vi "Read gRCP to Main.vi"(8 "error in (no error)":errorcluster, 11 "CIFTemplatePlugin in":refnum<class "TemplatePlugin.lvclass">) -> (0 "error out":errorcluster, 3 "CIFTemplatePlugin out":refnum<class "TemplatePlugin.lvclass">)   [LabVIEW 2021, in "TemplatePlugin.lvclass"]
uses:
  TemplatePlugin.lvclass
  TemplatePlugin.lvclass/TemplatePlugin.ctl
  CIF-LVCore/src/CIFUtilities/CIFOutOfBand/CIFOutOfBand.lvclass/CIFOutOfBand.ctl
  OOB/OOB_Rx/Private/Read Payload.vi
  CIF-LVCore/src/CIFUtilities/CIFOutOfBand/Read OOB DVR.vi
  OOB/OOB_Rx/Private/Command Settings.vi
  CIF-LVCore/src/CIFUtilities/CIFOutOfBand/Accessors/Read Local OOB Data.vi
  OOB/OOB_Rx/TemplateOOB_Rx.lvclass
  D:/dev/CIF-LVCore/src/CIFUtilities/CIFOutOfBand/CIFOutOfBand.lvclass
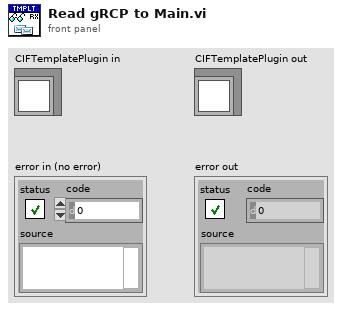
[diagram p1: front panel]
types:
  T1 = typedef "TemplateOOB_Rx.lvclass/OOB Commands.ctl" = enum8{"Command 1"}
  T2 = typedef "TemplateOOB_Rx.lvclass/gRPC to Main Command Data.ctl" = cluster{"Cmd 1 Data":i32}
  T3 = typedef "TemplatePlugin.lvclass/gRPC to Main Cyclic Data.ctl" = cluster{"Cyclic Data 1":i32}
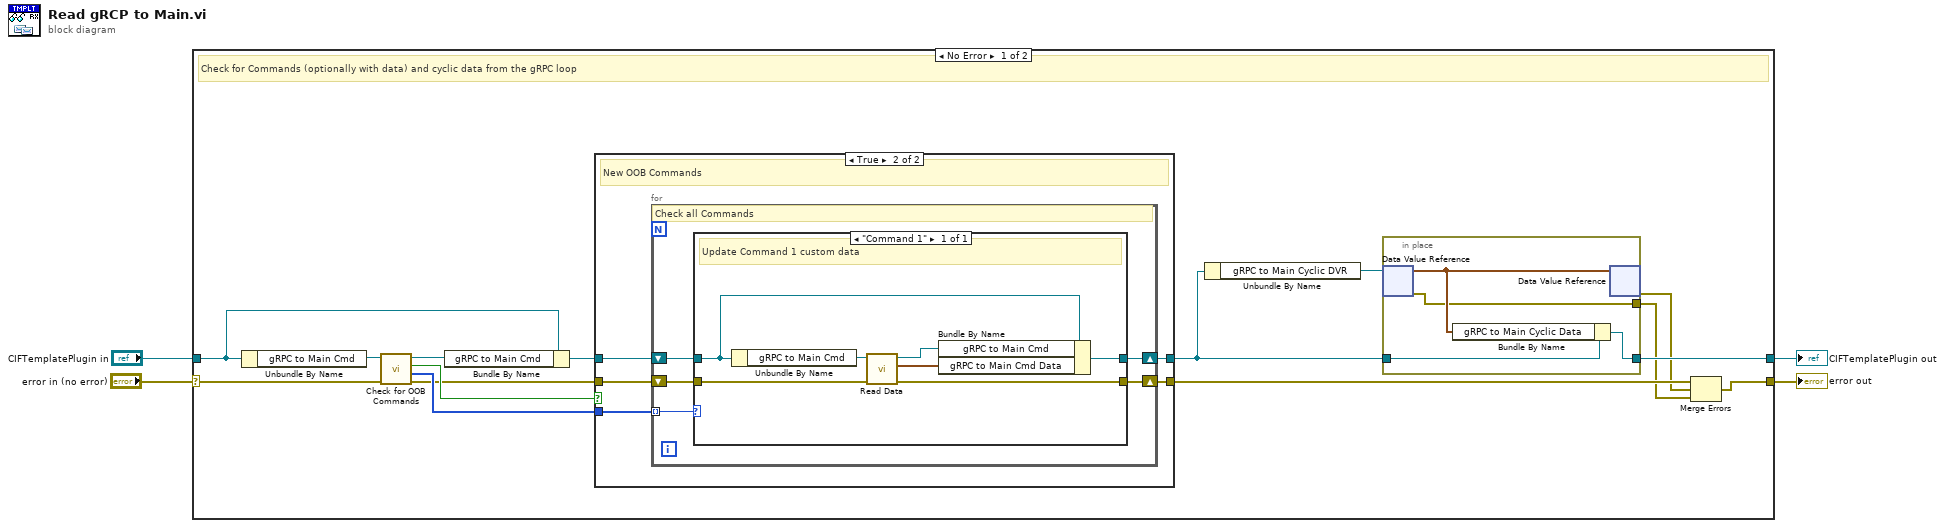
[diagram p0: block diagram]
diagram:
  n1 = case shown="No Error" "error in (no error)" {
    selector: "error in (no error)" -> [w19 w44]
    tunnel: [w12 w44] -> w3
    tunnel: [w14 w43] -> w1
    tunnel: "CIFTemplatePlugin in" -> [w7 w43]
    frame No Error {
      # "Check for Commands (optionally with data) and cyclic data from the gRPC loop"
      n2 = Unbundle By Name(w7) -> ("gRPC to Main Cmd"=w9:refnum<class "TemplateOOB_Rx.lvclass">)
      n3 = call "Check for OOB Commands.vi"("error in (no error)"=w19, "CoreOOB_Rx in"=w9) -> ("error out"=w16:errorcluster, "Commands"=w17:T1[], "New Commands"=w18:bool, "CoreOOB_Rx out"=w8:refnum<class "TemplateOOB_Rx.lvclass">)  [unwired: 6 in]
      n4 = Bundle By Name(cluster=w7, "gRPC to Main Cmd"=w8) -> (w6:refnum<class "TemplatePlugin.lvclass">)
      n5 = case shown="True" w18 {
        tunnel: w17 -> [_ w30]
        tunnel: w6 -> [w25 w29]
        tunnel: [w25 w27] -> w5
        tunnel: w16 -> [w24 w28]
        tunnel: [w24 w26] -> w13
        frame False {
          # "No new OOB Commands"
        }
        frame True {
          # "New OOB Commands"
          n6 = for {
            tunnel: w30 -> [w35] mode=indexing
            shift-right: [w32] -> w27
            shift-left: w29 -> [w33]
            shift-right: [w31] -> w26
            shift-left: w28 -> [w34]
            # "Check all Commands"
            n7 = case shown="\"Command 1\"" w35 {
              tunnel: w34 -> [w42]
              tunnel: w33 -> [w39]
              tunnel: [w38] -> w32
              tunnel: [w41] -> w31
              frame "Command 1" {
                # "Update Command 1 custom data"
                n8 = Unbundle By Name(w39) -> ("gRPC to Main Cmd"=w40:refnum<class "TemplateOOB_Rx.lvclass">)
                n9 = call "Read Data.vi"("error in"=w42, "CutomOOB_Rx in"=w40) -> ("error out"=w41:errorcluster, "Data"=w36:T2, "CutomOOB_Rx out"=w37:refnum<class "TemplateOOB_Rx.lvclass">)  [unwired: 7 in]
                n10 = Bundle By Name(cluster=w39, "gRPC to Main Cmd"=w37, "gRPC to Main Cmd Data"=w36) -> (w38:refnum<class "TemplatePlugin.lvclass">)
              }
            }
          }
        }
      }
      n11 = Unbundle By Name(w5) -> ("gRPC to Main Cyclic DVR"=w15:refnum<data-value>)
      n12 = in-place {
        in-place-border: w5 -> [w23]
        in-place-border: [w21] -> w14
        in-place-border: [w20] -> w10
        n13 = in-place-dvr #1(w15) -> (w22:T3, w20:errorcluster)
        n14 = Bundle By Name(cluster=w23, "gRPC to Main Cyclic Data"=w22) -> (w21:refnum<class "TemplatePlugin.lvclass">)
        n15 = in-place-dvr #1(w22) -> (w11:errorcluster)  [unwired: 1 out]
      }
      n16 = Merge Errors(w13, w11, w10) -> (w12:errorcluster)
    }
    frame Error {
    }
  }
  "error out" <- w3
  "CIFTemplatePlugin out" <- w1
